vi "ALONE_EUROTHERM.vi"(7 "Refresco(s)":dbl=5.0 caption="Elapsed Time (s)", 8 "error in (no error)":errorcluster) -> (0 "Error Out":errorcluster, 5 "Remote?":bool)   [LabVIEW 2017]
uses:
  EUROTHERM/2xP116.ctl
  EUROTHERM/TEG P116x2w.ctl
  <vilib>/Utility/error.llb/DialogType.ctl
  EUROTHERM/Eurotherm_2023_Module.ctl
  SERIAL RASP_PICO VALVE/kissia_rasPico Module.ctl
  REACTOR_GLOBALES.vi
panel:
  out "MaxOut":T1
  out "VALVE.":bool
  in  "VALVE":bool
  out "Potencia":T1
  in  "SP":bool
  out "ERROR":bool
  out "P116x2":T2
  out "TargetSP(C)":T1
  out "WorkingSP(C)":T1
  out "TempPV(C)":T1
  in  "Write":bool
  out "RateSP(C/min)":T1
  out "ERRORES":i32=5 caption="Elapsed Time (s)"
  out "Time (m)":dbl caption="Elapsed Time (s)" format="%.1f"
  out "Date":string caption="asd"
  out "Time":string caption="asd"
  in  "Refres":bool
  out "CICLO":i32=5 caption="Elapsed Time (s)"
  in  "stop":bool
  # "Control temperatura"
  # "Eurotherm P116"
  # "CALOR"
  # "FRIO"
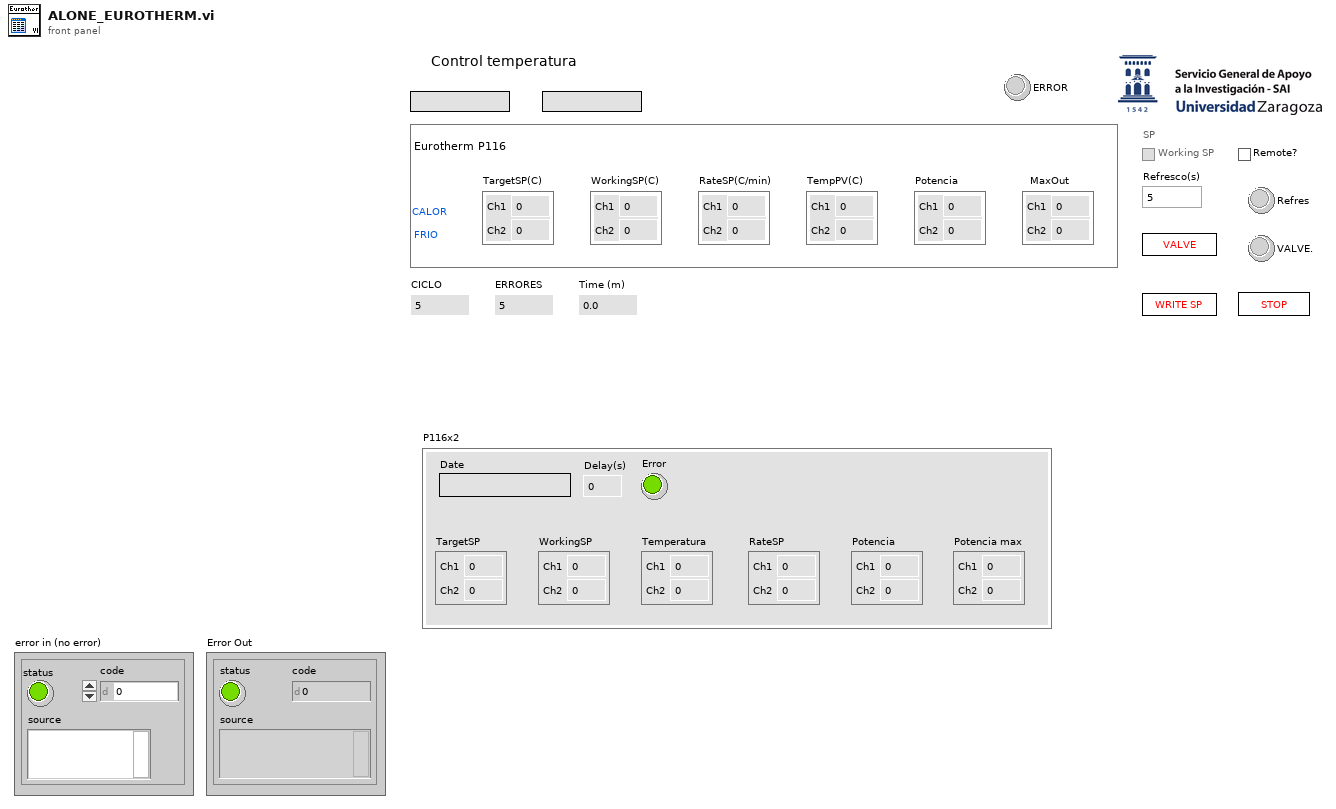
[diagram p1: front panel]
types:
  T1 = typedef "2xP116.ctl" = cluster{"Ch1":dbl, "Ch2":dbl}
  T2 = typedef "TEG P116x2w.ctl" = cluster{"TargetSP":T1, "WorkingSP":T1, "Temperatura":T1, "Error":bool, "Date":string, "Delay(s)":dbl, "RateSP":T1, "Potencia":T1, "Potencia max":T1}
  T3 = typedef "kissia_rasPico Module.ctl" = enum16{"Initialize", "Read Data", "Write Data", "Enable", "Disable", "Shutdown"}
  T4 = typedef "Eurotherm_2023_Module.ctl" = enum16{"Initialize", "Write setpoint", "Read data", "Write ramp rate", "Set constante proporcional", "Set constante integral", "Set constante diferencial", "Set ouput limit LOW", "Set ouput limit HIGH", "Shutdown"}
  T5 = typedef "DialogType.ctl" = u16
  T6 = typedef "REACTOR_COMUNICACIONES.ctl" = cluster{"Alicats":refnum<visa-resource-name>, "Alic":bool, "eValve":refnum<visa-resource-name>, "eval":bool, "Eurotherm":refnum<visa-resource-name>, "euro":bool, "Cell GAS":refnum<visa-resource-name>, "cgas":bool, "Cell H2S":refnum<visa-resource-name>, "ch2s":bool}
  T7 = enum16{"Add 1", "Add 2", "Add 3", "Add 10", "Add 11", "Add 12", "Add 13"}[]
  T8 = cluster{"processVal":dbl, "targetSP":dbl, "workingSP":dbl, "workingOut":dbl}
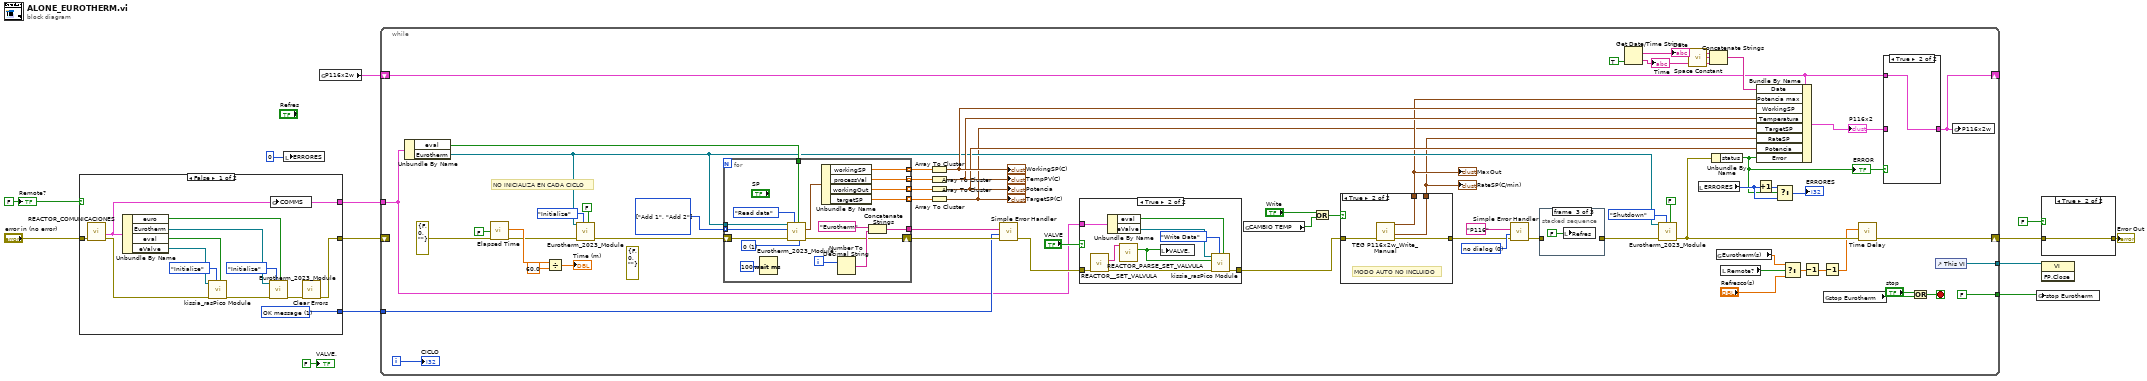
[diagram p0: block diagram]
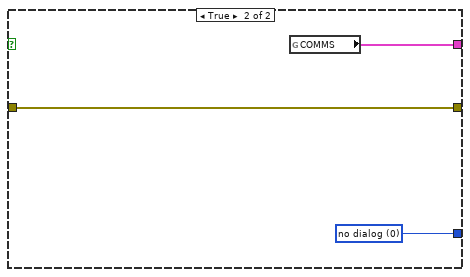
[diagram p3: hidden frame]
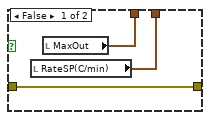
[diagram p6: hidden frame]
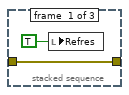
[diagram p7: hidden frame]
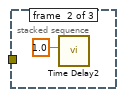
[diagram p8: hidden frame]
diagram:
  w11 = FALSE ("Remote?")
  n1 = case shown="False" w11 {
    tunnel: [w23 w29] -> w9
    tunnel: "error in (no error)" -> [w26 w28]
    tunnel: [w19 w28] -> w3
    tunnel: [w25 w27] -> w4
    frame False {
      w25 = T5 1 items=["no dialog", "OK message", "continue or stop message", "OK message + warnings", "continue/stop + warnings"] ("type of dialog (OK msg:1)")
      n2 = call "REACTOR_COMUNICACIONES.vi"("error in (no error)"=w26) -> ("error out"=w17:errorcluster, "COMMS"=w23:T6)  [unwired: 8 in, 1 out]
      n3 = Unbundle By Name(w23) -> ("euro"=w22:bool, "Eurotherm"=w21:refnum<visa-resource-name>, "eval"=w14:bool, "eValve"=w15:refnum<visa-resource-name>)
      n4 = call "kissia_rasPico Module.vi"("Enable"=w14, "Command"=kissia_rasPico_Module."Initialize", "error in (no error)"=w17, "VISA resource name"=w15) -> ("error out"=w16:errorcluster)  [unwired: 4 in, 3 out]
      n5 = call "Eurotherm_2023_Module.vi"("Eurotherm (T:Enable)"=w22, "Command"=Eurotherm_2023_Module."Initialize", "error in (no error)"=w16, "VISA resource name"=w21) -> ("error out"=w20:errorcluster)  [unwired: 6 in, 1 out]
      n6 = global write "REACTOR_GLOBALES.vi" "COMMS"(w23) -> ()
      n7 = call <vilib>:"Clear Errors.vi"("error in (no error)"=w20) -> ("error out"=w19:errorcluster)  [unwired: 5 in, 1 out]
    }
    frame True {
      w27 = T5 0 items=["no dialog", "OK message", "continue or stop message", "OK message + warnings", "continue/stop + warnings"] ("type of dialog (OK msg:1)")
      n8 = global read "REACTOR_GLOBALES.vi" "COMMS"() -> (w29:T6)
    }
  }
  n9 = local write "ERRORES"(0 ("Errores")) -> ()
  n10 = global read "REACTOR_GLOBALES.vi" "P116x2w"() -> (w2:T2)
  n11 = while {
    shift-right: [w41] -> w6
    shift-left: w3 -> [_]
    tunnel: [FALSE ("stop")] -> w13
    tunnel: [w82] -> w12
    tunnel: w9 -> [w35]
    tunnel: w4 -> [w60]
    shift-right: [w62] -> _
    shift-left: w2 -> [w58]
    i -> [w46]
    stop <- w91 stop-if-true
    (unwired) errorcluster {"status"=FALSE, "code"=0, "source"=""} ("error in (no error)")
    w71 = T7 [enum."Add 1", enum."Add 2"] items=["Add 1", "Add 2", "Add 3", "Add 10", "Add 11", "Add 12", "Add 13"]
    w73 = T5 0 items=["no dialog", "OK message", "continue or stop message", "OK message + warnings", "continue/stop + warnings"] ("type of dialog (OK msg:1)")
    # "NO INICIALIZA EN CADA CICLO"
    n12 = Unbundle By Name(w35) -> ("eval"=w47:bool, "Eurotherm"=w40:refnum<visa-resource-name>)
    n13 = call "Elapsed Time"("Auto Reset"=FALSE, "error in (no error)"=errorcluster {"status"=FALSE, "code"=0, "source"=""}) -> ("Elapsed Time (s)"=w88:dbl, "error out"=w49:errorcluster)  [unwired: 10 in, 6 out]
    n14 = Divide(x=w88, y=60.0) -> (x/y=→"Time (m)":dbl)
    n15 = call "Eurotherm_2023_Module.vi"("Eurotherm (T:Enable)"=FALSE, "Command"=Eurotherm_2023_Module."Initialize", "error in (no error)"=w49, "VISA resource name"=w40) -> ("error out"=w50:errorcluster)  [unwired: 6 in, 1 out]
    n16 = for {
      tunnel: w71 -> [w108] mode=indexing
      tunnel: [w112] -> w70 mode=indexing
      tunnel: [w111] -> w69 mode=indexing
      shift-right: [w117] -> w64
      shift-left: w50 -> [w118]
      tunnel: w47 -> [w116]
      tunnel: [w120] -> w63
      tunnel: w40 -> [w115]
      tunnel: [w110] -> w54 mode=indexing
      tunnel: [w107] -> w33 mode=indexing
      i -> [w114]
      w109 = u16 1 items=["0"=1, "1"=10, "2"=100] ("Decimales")
      n17 = Wait (ms)(milliseconds to wait=u32 100) -> ()  [unwired: 1 out]
      n18 = call "Eurotherm_2023_Module.vi"("Decimales"=w109, "Eurotherm (T:Enable)"=w116, "Command"=Eurotherm_2023_Module."Read data", "error in (no error)"=w118, "Address"=w108, "VISA resource name"=w115) -> ("error out"=w117:errorcluster, "Eurotherm"=w113:T8)  [unwired: 4 in]
      n19 = Unbundle By Name(w113) -> ("workingSP"=w112:dbl, "processVal"=w111:dbl, "workingOut"=w110:dbl, "targetSP"=w107:dbl)
      n20 = Number To Decimal String(number=w114) -> (decimal integer string=w121:string)  [unwired: 1 in]
      n21 = Concatenate Strings("Eurotherm" ("error source (\" \")"), w121) -> (w120:string)
    }
    n22 = Array To Cluster(array=w70) -> (cluster=w68:cluster{"[0]":dbl, "[1]":dbl})
    "WorkingSP(C)" <- w68
    n23 = Array To Cluster(array=w69) -> (cluster=w67:cluster{"[0]":dbl, "[1]":dbl})
    "TempPV(C)" <- w67
    n24 = Array To Cluster(array=w54) -> (cluster=w53:cluster{"[0]":dbl, "[1]":dbl})
    "Potencia" <- w53
    n25 = Array To Cluster(array=w33) -> (cluster=w31:cluster{"[0]":dbl, "[1]":dbl})
    "TargetSP(C)" <- w31
    n26 = call <vilib>:"Simple Error Handler.vi"("error source (\" \")"=w63, "type of dialog (OK msg:1)"=w60, "error in (no error)"=w64) -> ("error out"=w37:errorcluster)  [unwired: 2 in, 4 out]
    n27 = case shown="True" "VALVE" {
      tunnel: w37 -> [w95 w98]
      tunnel: [w95 w97] -> w36
      tunnel: w35 -> [_ w96]
      frame False {
      }
      frame True {
        n28 = call "REACTOR__SET_VALVULA.vi"("error in (no error)"=w98) -> ("error out"=w102:errorcluster, "resulting string 1"=w101:string)  [unwired: 6 in, 1 out]
        n29 = Unbundle By Name(w96) -> ("eval"=w99:bool, "eValve"=w103:refnum<visa-resource-name>)
        n30 = call "REACTOR_PARSE_SET_VALVULA.vi"("String"=w101) -> ("VALVULA 1"=w104:bool)  [unwired: 9 in, 1 out]
        n31 = local write "VALVE."(w104) -> ()
        n32 = call "kissia_rasPico Module.vi"("Enable"=w99, "Command"=kissia_rasPico_Module."Write Data", "error in (no error)"=w102, "VALVE"=w104, "VISA resource name"=w103) -> ("error out"=w97:errorcluster)  [unwired: 3 in, 3 out]
      }
    }
    n33 = global read "REACTOR_GLOBALES.vi" "CAMBIO TEMP"() -> (w56:bool)
    n34 = Or(x="Write", y=w56) -> (x .or. y?=w57:bool)
    n35 = case shown="True" w57 {
      tunnel: w36 -> [w126 w130]
      tunnel: [w126 w129] -> w55
      tunnel: [w125 w128] -> w32
      tunnel: [w124 w127] -> w30
      frame False {
        n36 = local read "RateSP(C/min)"() -> (w124:T1)
        n37 = local read "MaxOut"() -> (w125:T1)
      }
      frame True {
        # "MODO AUTO NO INCLUIDO"
        n38 = call "TEG P116x2w_Write_Manual.vi"("error in (no error)"=w130) -> ("error out"=w129:errorcluster, "RateSP(C/min) 2"=w127:T1, "MaxOutput 2"=w128:T1)  [unwired: 7 in, 1 out]
      }
    }
    "MaxOut" <- w32
    "RateSP(C/min)" <- w30
    n39 = call <vilib>:"Simple Error Handler.vi"("error source (\" \")"="P116" ("error source (\" \")"), "type of dialog (OK msg:1)"=w73, "error in (no error)"=w55) -> ("error out"=w65:errorcluster)  [unwired: 2 in, 4 out]
    n40 = stacked-sequence {
      tunnel: w65 -> [w131 _ _]
      tunnel: [w131 _ _] -> w42
      frame #0 {
        n41 = local write "Refres"(TRUE ("Refresh")) -> ()
      }
      frame #1 {
        n42 = call "Time Delay2"("Delay Time (s)"=1.0) -> ()  [unwired: 10 in, 1 out]
      }
      frame #2 {
        n43 = local write "Refres"(FALSE ("Refresh")) -> ()
      }
    }
    n44 = Get Date/Time String(want seconds? (F)=TRUE) -> (date string=w85:string, time string=w86:string)  [unwired: 2 in]
    "Time" <- w86
    "Date" <- w85
    n45 = call "Eurotherm_2023_Module.vi"("Eurotherm (T:Enable)"=FALSE, "Command"=Eurotherm_2023_Module."Shutdown", "error in (no error)"=w42, "VISA resource name"=w40) -> ("error out"=w39:errorcluster)  [unwired: 6 in, 1 out]
    n46 = call <vilib>:"Space Constant.vi"() -> ("String"=w94:string)
    n47 = local read "ERRORES"() -> (w78:i32)
    n48 = Concatenate Strings(w85, w94, w86) -> (w66:string)
    n49 = Unbundle By Name(w39) -> ("status"=w51:bool)
    "ERROR" <- w51
    n50 = global read "REACTOR_GLOBALES.vi" "Eurotherm(s)"() -> (w81:dbl)
    n51 = local read "Remote?"() -> (w75:bool)
    n52 = Bundle By Name(cluster=w58, "Date"=w66, "Potencia max"=w32, "WorkingSP"=w68, "Temperatura"=w67, "TargetSP"=w31, "RateSP"=w30, "Potencia"=w53, "Error"=w51) -> (w59:T2)
    "P116x2" <- w59
    n53 = Increment(x=w78) -> (x+1=w77:i32)
    n54 = Select(t=w77, s=w51, f=w78) -> (s? t:f=→"ERRORES":i32)
    n55 = Select(t=w81, s=w75, f="Refresco(s)") -> (s? t:f=w79:dbl)
    n56 = Decrement(x=w79) -> (x-1=w61:dbl)
    n57 = Decrement(x=w61) -> (x-1=w34:dbl)
    n58 = global read "REACTOR_GLOBALES.vi" "stop Eurotherm"() -> (w84:bool)
    n59 = call "Time Delay"("error in (no error)"=w39, "Delay Time (s)"=w34) -> ("error out"=w41:errorcluster)  [unwired: 9 in]
    n60 = case shown="True" w51 {
      tunnel: w59 -> [w105 _]
      tunnel: [w105 w106] -> w62
      tunnel: w58 -> [_ w106]
      frame False {
      }
      frame True {
      }
    }
    n61 = Or(x="stop", y=w84) -> (x .or. y?=w91:bool)
    n62 = control-ref of="This VI"() -> (w82:refnum<vi>)
    n63 = global write "REACTOR_GLOBALES.vi" "P116x2w"(w62) -> ()
    "CICLO" <- w46
  }
  n64 = global write "REACTOR_GLOBALES.vi" "stop Eurotherm"(w13) -> ()
  n65 = case shown="True" FALSE {
    tunnel: w6 -> [w135 w136]
    tunnel: [w135 w136] -> w5
    frame False {
    }
    frame True {
    }
  }
  "Error Out" <- w5
  n66 = invoke class="VI" method="FP.Close"(reference=w12) -> ()  [unwired: 2 in, 3 out]
  "Remote?" <- w11
  "VALVE." <- FALSE ("VALVE 2")
